vi "print_lua.vi"(5 "LuaVIEW reference in":T1) -> (15 "error out":errorcluster)   [LabVIEW 2012]
doc: "Print a line of text. Takes the provided arguments and converts them to printable strings. The resulting strings are concatenated with spaces inserted between strings and a linefeed appended to the end. The resulting line of text is then output to a floating console window which is opened and moved to front if not already so. All scripts using this function share the same console window so that output can get mixed up. The console history has a limited capacity (40000 characters).\n\nThe arguments can be of any type, but only the basic datatypes (boolean, number, and string) result in easily interpretable output. The content of functions and tables is not printed, only their unique reference pointers are printed as hexadecimal numbers. When no arguments are specified, only a linefeed will be printed.\nParameters:\n[any:arg], argument to be printed.\n..."
uses:
  typedefs/t_LuaVIEW Reference.ctl
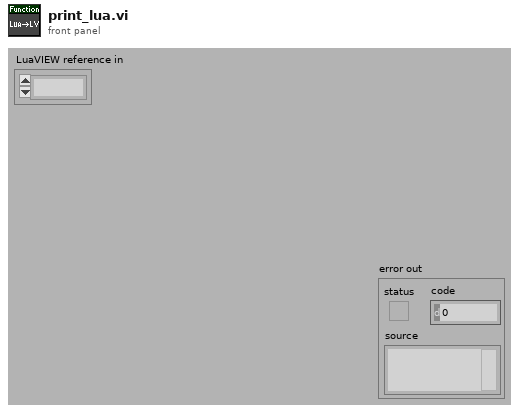
[diagram p1: front panel]
types:
  T1 = typedef "t_LuaVIEW Reference.ctl" = refnum<k1>
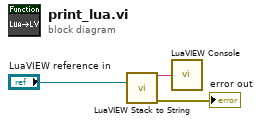
[diagram p0: block diagram]
diagram:
  n1 = call "LuaVIEW Stack to String.vi"("LuaVIEW reference in"="LuaVIEW reference in") -> ("string"=w2:string, "error out"=→"error out":errorcluster)  [unwired: 12 in, 1 out]
  n2 = call "LuaVIEW Console.vi"("print string"=w2) -> ()  [unwired: 1 in]
